vi "E11_Demo_M_Garcia_Denise.vi"() -> ()   [LabVIEW 2017]
uses:
  <vilib>/Analysis/baseanly.llb/Mean (DBL).vi
  <vilib>/Analysis/NI_AALBase.lvlib
panel:
  out "Velocity (m/s)":dbl format="%0.2f"
  in  "Voltage":dbl(slide) scale=0.0..10.0
  in  "Transducer Offset [V]":dbl
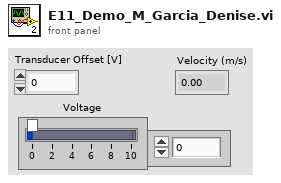
[diagram p1: front panel]
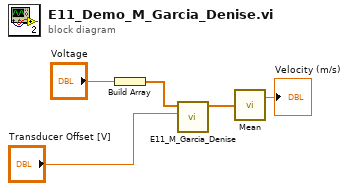
[diagram p0: block diagram]
diagram:
  n1 = Build Array("Voltage") -> (w4:dbl[])
  n2 = call "E11_M_Garcia_Denise.vi"("Transducer Offset [V]"="Transducer Offset [V]", "Voltage Input [m/s]"=w4) -> ("Velocity Output [m/s]"=w2:dbl[])  [unwired: 9 in]
  n3 = call-poly <vilib>:"Mean.vi"("X"=w2) -> ("mean"=→"Velocity (m/s)":dbl)  [unwired: 1 out]
